vi "WriteData.vi"(2 "error in":errorcluster, 3 "Log data":T1, 4 "File handle":refnum<file>) -> (0 "error out":errorcluster, 1 "File handle out":refnum<file>)   [LabVIEW 2015]
doc: "Write a timestamp and a series of floats to the given file, seperated by tabs and terminated by a newline."
panel:
  out "Output string":string
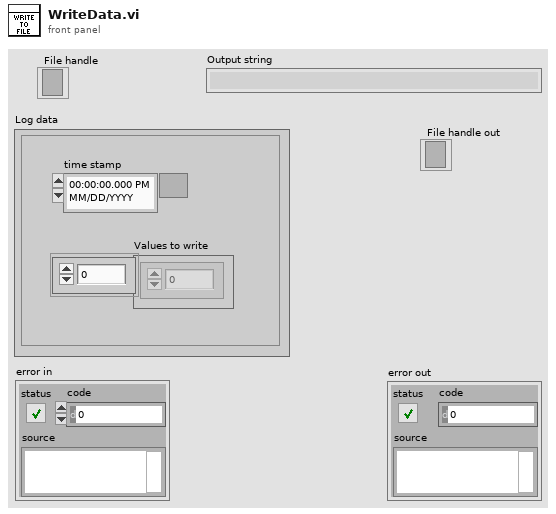
[diagram p1: front panel]
types:
  T1 = cluster{"time stamp":timestamp, "Values to write":dbl[]}
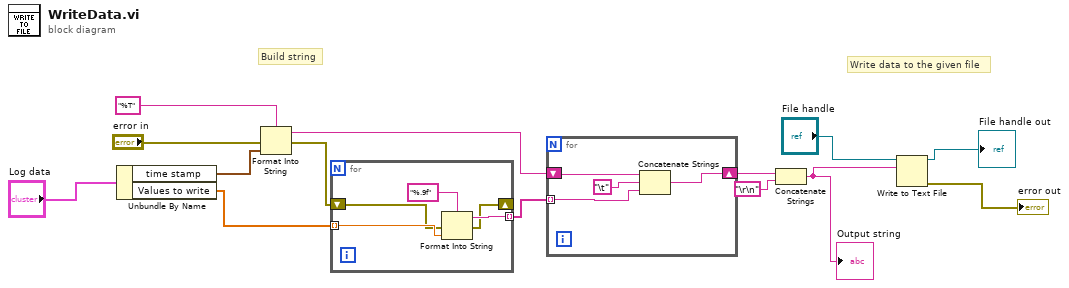
[diagram p0: block diagram]
diagram:
  # "Build string"
  # "Write data to the given file"
  n1 = Unbundle By Name("Log data") -> ("time stamp"=w10:timestamp, "Values to write"=w7:dbl[])
  n2 = Format Into String(format string="%T", error in="error in", w10) -> (resulting string=w5:string, error out=w1:errorcluster)  [unwired: 1 in]
  n3 = for {
    tunnel: w7 -> [w18] mode=indexing
    tunnel: [w17] -> w6 mode=indexing
    shift-right: [w15] -> _
    shift-left: w1 -> [w16]
    n4 = Format Into String(format string="%.9f", error in=w16, w18) -> (resulting string=w17:string, error out=w15:errorcluster)  [unwired: 1 in]
  }
  n5 = for {
    tunnel: w6 -> [w21] mode=indexing
    shift-right: [w20] -> w4
    shift-left: w5 -> [w23]
    n6 = Concatenate Strings(w23, "\t", w21) -> (w20:string)
  }
  n7 = Concatenate Strings(w4, "\r\n") -> (w2:string)
  "Output string" <- w2
  n8 = Write to Text File(file (use dialog)="File handle", text=w2) -> (refnum out=→"File handle out":refnum<file>, error out=→"error out":errorcluster)  [unwired: 2 in, 1 out]
